vi "Round Voltages.vi"(2 "Rouding Factor (0.001 volts)":T2(ring), 7 "ADC Readings (rounded)":T1) -> (8 "ADC Readings (rounded)":T1)   [LabVIEW 2017]
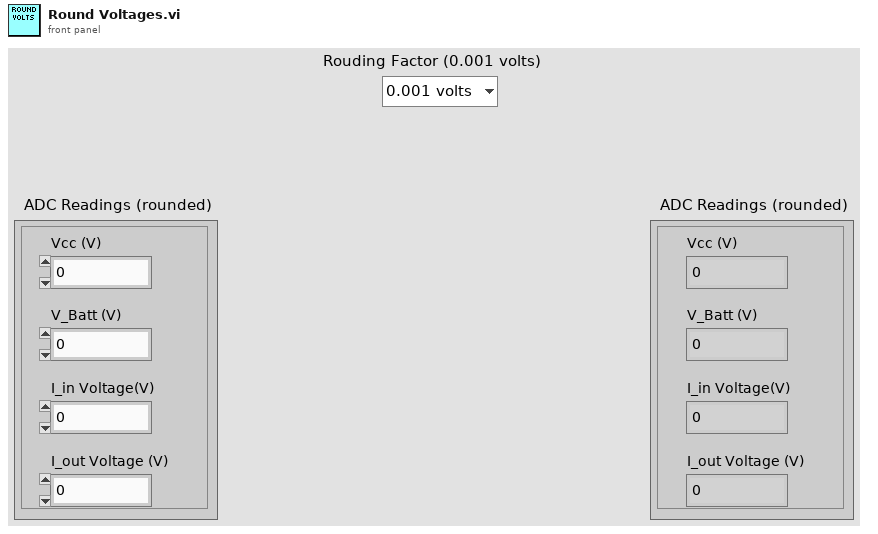
[diagram p1: front panel]
types:
  T1 = cluster{"Vcc (V)":dbl, "V_Batt (V)":dbl, "I_in Voltage(V)":dbl, "I_out Voltage (V)":dbl}
  T2 = enum16{"0.001 volts", "0.01 volts", "0.1 volts", "1 volt"}
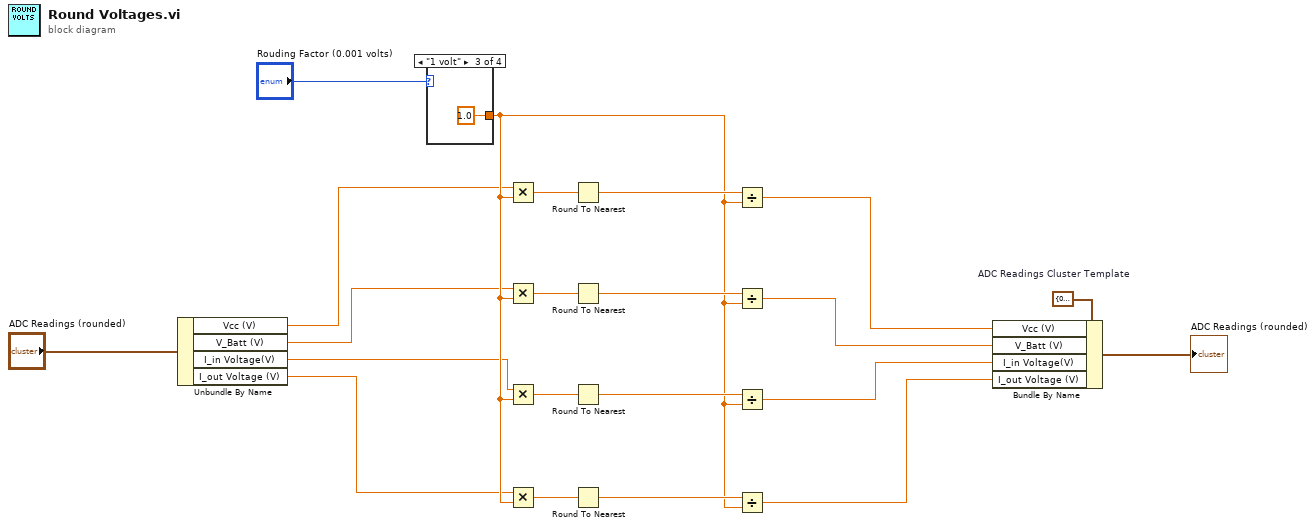
[diagram p0: block diagram]
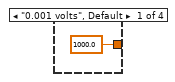
[diagram p2: hidden frame]
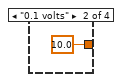
[diagram p3: hidden frame]
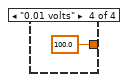
[diagram p4: hidden frame]
diagram:
  w3 = T1 {"Vcc (V)"=0.0, "V_Batt (V)"=0.0, "I_in Voltage(V)"=0.0, "I_out Voltage (V)"=0.0}  # ADC Readings Cluster Template
  n1 = Unbundle By Name("ADC Readings (rounded)") -> ("Vcc (V)"=w11:dbl, "V_Batt (V)"=w10:dbl, "I_in Voltage(V)"=w9:dbl, "I_out Voltage (V)"=w8:dbl)
  n2 = case shown="\"1 volt\"" "Rouding Factor (0.001 volts)" {
    tunnel: [1000.0 ("x") 10.0 ("x") 1.0 ("x") 100.0 ("x")] -> w12
    frame "0.001 volts", Default {
    }
    frame "0.1 volts" {
    }
    frame "1 volt" {
    }
    frame "0.01 volts" {
    }
  }
  n3 = Multiply(x=w11, y=w12) -> (x*y=w21:dbl)
  n4 = Multiply(x=w10, y=w12) -> (x*y=w18:dbl)
  n5 = Multiply(x=w9, y=w12) -> (x*y=w16:dbl)
  n6 = Multiply(x=w8, y=w12) -> (x*y=w14:dbl)
  n7 = Round To Nearest(number=w21) -> (nearest integer value=w20:dbl)
  n8 = Round To Nearest(number=w18) -> (nearest integer value=w17:dbl)
  n9 = Round To Nearest(number=w16) -> (nearest integer value=w15:dbl)
  n10 = Round To Nearest(number=w14) -> (nearest integer value=w13:dbl)
  n11 = Divide(x=w20, y=w12) -> (x/y=w7:dbl)
  n12 = Divide(x=w17, y=w12) -> (x/y=w6:dbl)
  n13 = Divide(x=w15, y=w12) -> (x/y=w5:dbl)
  n14 = Divide(x=w13, y=w12) -> (x/y=w4:dbl)
  n15 = Bundle By Name(cluster=w3, "Vcc (V)"=w7, "V_Batt (V)"=w6, "I_in Voltage(V)"=w5, "I_out Voltage (V)"=w4) -> (→"ADC Readings (rounded)":T1)
